vi "reallocate_buffers.vi"(8 "error in (no error)":errorcluster, 11 "ImageAssemblerRK110612Spiral in":refnum<class "ImageAssemblerRK110612Spiral.lvclass">) -> (0 "error out":errorcluster, 3 "ImageAssemblerRK110612Spiral out":refnum<class "ImageAssemblerRK110612Spiral.lvclass">)   [LabVIEW 2010, in "ImageAssemblerRK110612Spiral.lvclass"]
uses:
  ImageAssemblerRK110612Spiral.lvclass
  ImageAssemblerRK110612Spiral.lvclass/ImageAssemblerRK110612Spiral.ctl
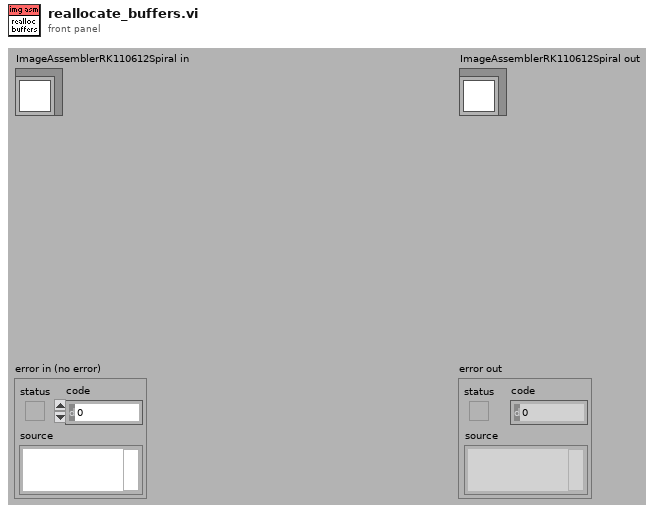
[diagram p1: front panel]
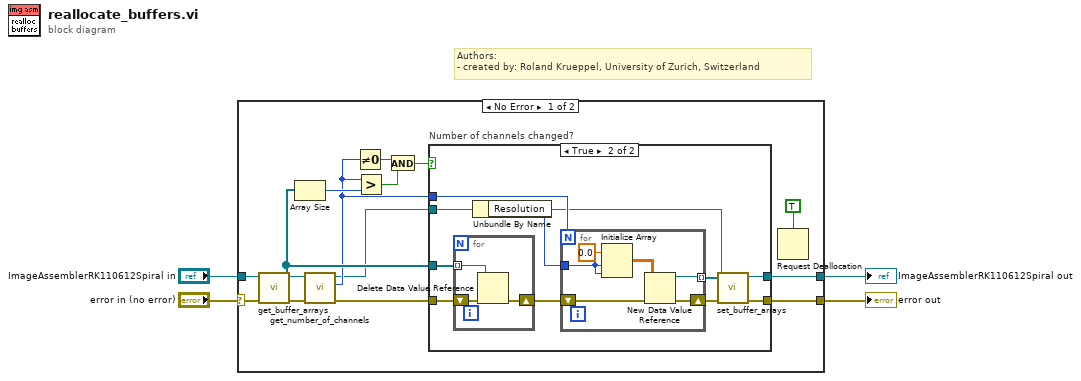
[diagram p0: block diagram]
diagram:
  # "Authors: \n- created by: Roland Krueppel, University of Zurich, Switzerland"
  n1 = case shown="No Error" "error in (no error)" {
    selector: "error in (no error)" -> [w7 w42]
    tunnel: [w6 w42] -> w3
    tunnel: [w8 w41] -> w1
    tunnel: "ImageAssemblerRK110612Spiral in" -> [w9 w41]
    frame No Error {
      n2 = call-dynamic "get_buffer_arrays.vi"("error in (no error)"=w7, "ImageAssemblerRK110612Spiral in"=w9) -> ("error out"=w17:errorcluster, "Buffer arrays"=w12:refnum<data-value>[], "ImageAssemblerRK110612Spiral out"=w16:refnum<class "ImageAssemblerRK110612Spiral.lvclass">)  [unwired: 7 in]
      n3 = Array Size(array=w12) -> (size(s)=w15:i32)
      n4 = call-dynamic "get_number_of_channels.vi"("error in (no error)"=w17, "GenericImageAssembler.lvclass in"=w16) -> ("error out"=w13:errorcluster, "number of channels"=w11:i32, "GenericImageAssembler.lvclass out"=w10:refnum<class "ImageAssemblerRK110612Spiral.lvclass">)  [unwired: 7 in]
      n5 = Not Equal To 0?(x=w11) -> (x != 0?=w19:bool)
      n6 = Greater?(x=w11, y=w15) -> (0:w18:bool)
      n7 = And(x=w19, y=w18) -> (x .and. y?=w14:bool)
      n8 = case "Number of channels changed?" shown="True" w14 {
        tunnel: w13 -> [w21 w31]
        tunnel: w12 -> [_ w30]
        tunnel: w11 -> [_ w28]
        tunnel: w10 -> [w20 w26]
        tunnel: [w21 w22] -> w6
        tunnel: [w20 w23] -> w8
        frame False {
        }
        frame True {
          n9 = for {
            tunnel: w30 -> [w40] mode=indexing
            shift-right: [w38] -> w29
            shift-left: w31 -> [w39]
            n10 = Delete Data Value Reference(data value reference=w40, error in=w39) -> (error out=w38:errorcluster)  [unwired: 1 out]
          }
          n11 = Unbundle By Name(w26) -> ("Resolution"=w27:i32)
          n12 = for {
            N: w28 -> [_]
            tunnel: w27 -> [w37]
            shift-right: [w33] -> w25
            shift-left: w29 -> [w34]
            tunnel: [w32] -> w24 mode=indexing
            n13 = Initialize Array(sgl 0.0 ("element"), w37, w37) -> (w35:sgl[][])
            n14 = New Data Value Reference(data value=w35, error in=w34) -> (data value reference=w32:refnum<data-value>, error out=w33:errorcluster)
          }
          n15 = call-dynamic "set_buffer_arrays.vi"("error in (no error)"=w25, "Buffer arrays"=w24, "ImageAssemblerRK110612Spiral in"=w26) -> ("error out"=w22:errorcluster, "ImageAssemblerRK110612Spiral out"=w23:refnum<class "ImageAssemblerRK110612Spiral.lvclass">)  [unwired: 7 in]
        }
      }
      n16 = Request Deallocation(TRUE ("flag")) -> ()
    }
    frame Error {
    }
  }
  "error out" <- w3
  "ImageAssemblerRK110612Spiral out" <- w1
